vi "Parse All Attributes.vi"(8 "error in":errorcluster, 11 "Node In":refnum<k20>) -> (0 "error out":errorcluster, 2 "Section Data":T1, 3 "Node out":refnum<k20>)   [LabVIEW 2024, in "Parser.lvlib" / "Section.lvclass"]
uses:
  Section.lvclass
  <vilib>/xml/Close Reference(Node).vi
  <resource>/objmgr/DOMUserDefRef.rc
  <vilib>/xml/NI_XML.lvlib
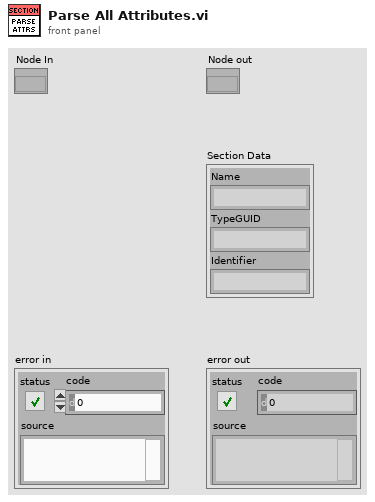
[diagram p1: front panel]
types:
  T1 = cluster{"Name":string, "TypeGUID":string, "Identifier":string}
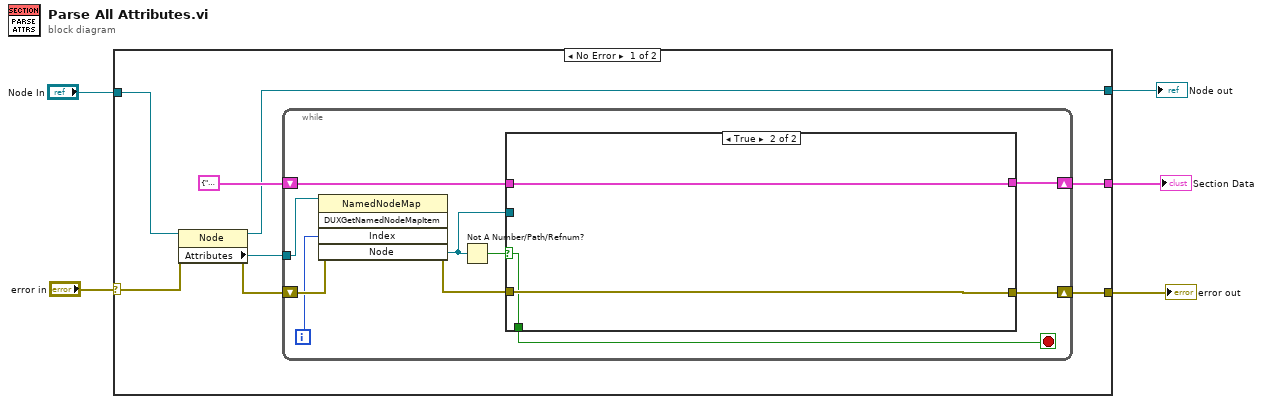
[diagram p0: block diagram]
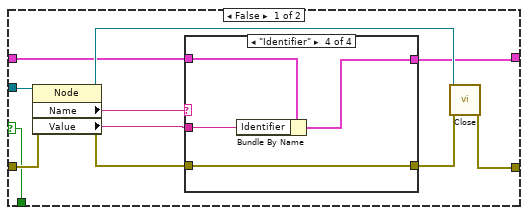
[diagram p2: hidden frame]
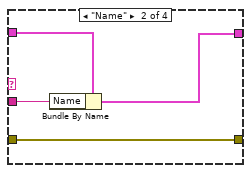
[diagram p4: hidden frame]
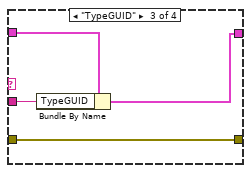
[diagram p5: hidden frame]
diagram:
  n1 = case shown="No Error" "error in" {
    selector: "error in" -> [w11 w53]
    tunnel: [w12 w53] -> w5
    tunnel: "Node In" -> [w10 w52]
    tunnel: [w7 w52] -> w2
    tunnel: [w6 _] -> w1
    frame No Error {
      n2 = property on="Property Node" class="Node"(reference=w10, error in=w11) -> (reference out=w7:refnum<k20>, error out=w13:errorcluster, "Attributes"=w9:refnum<k20>)
      n3 = while {
        tunnel: w9 -> [w20]
        shift-right: [w21] -> w12
        shift-left: w13 -> [w23]
        shift-right: [w14] -> w6
        shift-left: T1 {"Name"="", "TypeGUID"="", "Identifier"=""} ("Cluster of class private data") -> [w15]
        i -> [w18]
        stop <- w17 stop-if-true
        n4 = invoke on="Invoke Node" class="NamedNodeMap" method="DUXGetNamedNodeMapItem"(reference=w20, error in=w23, "Index"=w18) -> (error out=w22:errorcluster, "Node"=w16:refnum<k20>)  [unwired: 2 in, 3 out]
        n5 = Not A Number/Path/Refnum?(number/path/refnum=w16) -> (NaN/Path/Refnum?=w19:bool)
        n6 = case shown="True" w19 {
          selector: w19 -> [w28 w50]
          tunnel: w16 -> [w30 _]
          tunnel: w22 -> [w34 w51]
          tunnel: [w32 w51] -> w21
          tunnel: [w28 w50] -> w17
          tunnel: w15 -> [w25 w49]
          tunnel: [w24 w49] -> w14
          frame False {
            n7 = property on="Property Node" class="Node"(reference=w30, error in=w34) -> (reference out=w26:refnum<k20>, error out=w33:errorcluster, "Name"=w29:string, "Value"=w27:string)
            n8 = case shown="\"Identifier\"" w29 {
              tunnel: w27 -> [_ w39 w43 w47]
              tunnel: w33 -> [w36 w40 w44 w48]
              tunnel: w25 -> [w35 w38 w42 w46]
              tunnel: [w35 w37 w41 w45] -> w24
              tunnel: [w36 w40 w44 w48] -> w31
              frame "-1", Default {
              }
              frame "Name" {
                n9 = Bundle By Name(cluster=w38, "Name"=w39) -> (w37:T1)
              }
              frame "TypeGUID" {
                n10 = Bundle By Name(cluster=w42, "TypeGUID"=w43) -> (w41:T1)
              }
              frame "Identifier" {
                n11 = Bundle By Name(cluster=w46, "Identifier"=w47) -> (w45:T1)
              }
            }
            n12 = call-poly <vilib>:"Close.vi"("error in (no error)"=w31, "node"=w26) -> ("error out"=w32:errorcluster)  [unwired: 7 in]
          }
          frame True {
          }
        }
      }
    }
    frame Error {
    }
  }
  "error out" <- w5
  "Node out" <- w2
  "Section Data" <- w1
